vi "Arduino Find Home.vi"(7 "log ref":refnum<file>, 8 "error in":errorcluster, 9 "Homing Parameters":T1={"Direction (F: CW)"=FALSE, "Speed"=400, "Accel"=400, "Min Distance"=2700, "Short Leg"=0, "Error Cnts"=0}, 10 "Motor":i32, 11 "Addr":refnum<visa-resource-name>) -> (0 "error out":errorcluster, 2 "Success":bool, 3 "Log":string)   [LabVIEW 2021, in "FW Arduino Control.lvclass"]
uses:
  FW Arduino Control.lvclass
  Filter Wheel Arduino Homing cluster.ctl
panel:
  out "moves":i32
  out "Move distances":i32[](array[numeric])
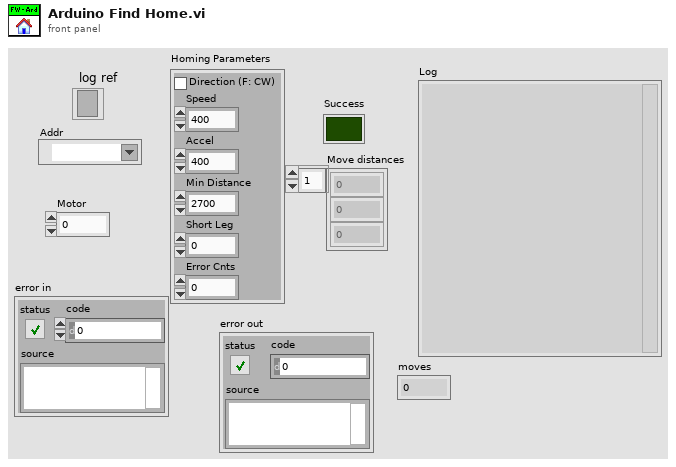
[diagram p1: front panel]
types:
  T1 = typedef "Filter Wheel Arduino Homing cluster.ctl" = cluster{"Direction (F: CW)":bool, "Speed":i32, "Accel":i32, "Min Distance":i32, "Short Leg":i32, "Error Cnts":i32}
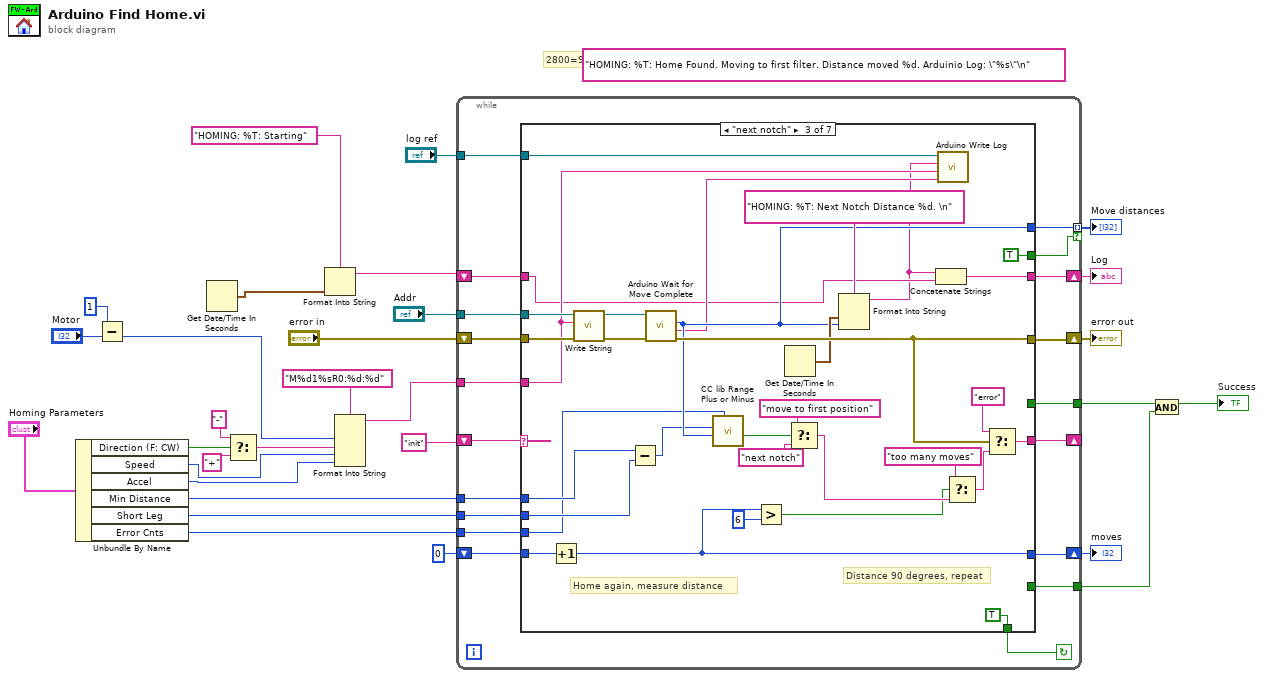
[diagram p0: block diagram]
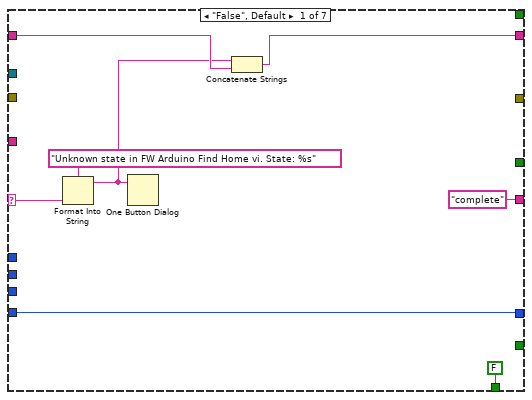
[diagram p2: hidden frame]
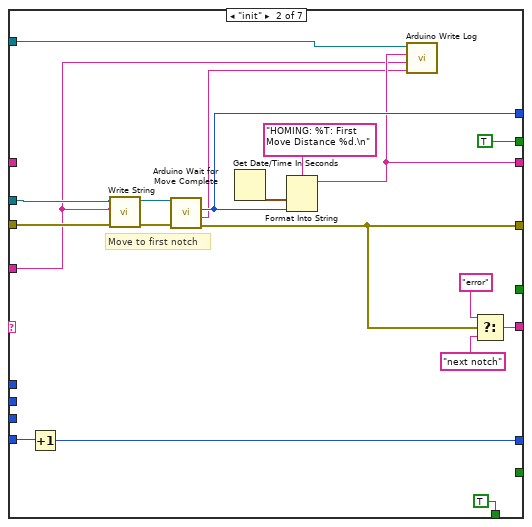
[diagram p3: hidden frame]
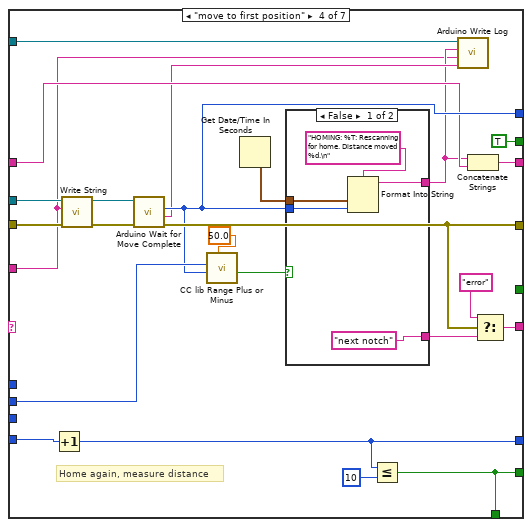
[diagram p4: hidden frame]
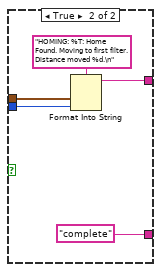
[diagram p5: hidden frame]
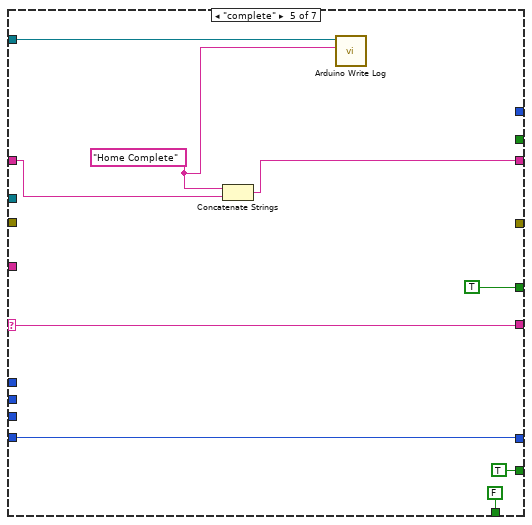
[diagram p6: hidden frame]
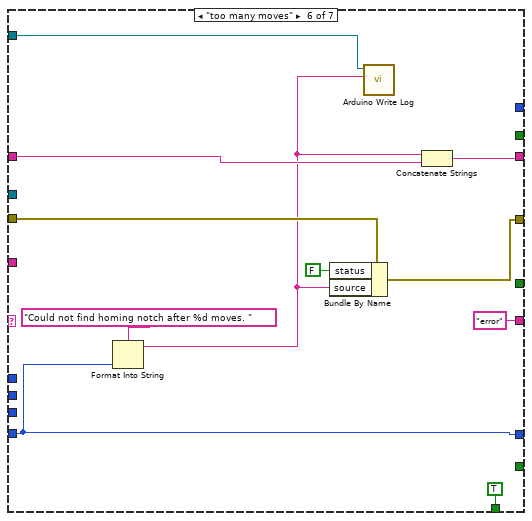
[diagram p7: hidden frame]
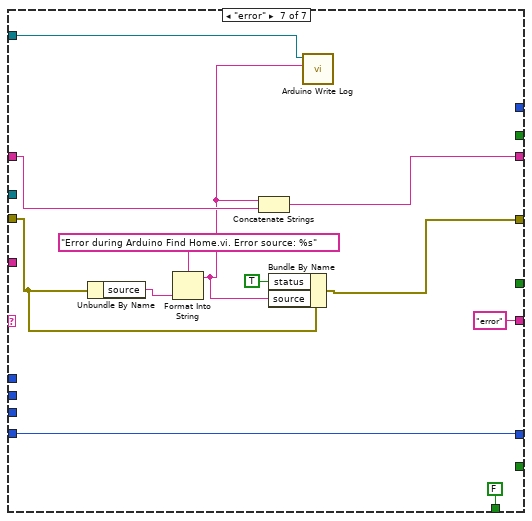
[diagram p8: hidden frame]
diagram:
  (unwired) "HOMING: %T: Home Found. Moving to first filter. Distance moved %d. Arduinio Log: \"%s\"\n" ("format string")
  # "2800=90degrees"
  n1 = Unbundle By Name("Homing Parameters") -> ("Direction (F: CW)"=w19:bool, "Speed"=w18:i32, "Accel"=w17:i32, "Min Distance"=w12:i32, "Short Leg"=w10:i32, "Error Cnts"=w1:i32)
  n2 = Subtract(x=1, y="Motor") -> (x-y=w3:i32)
  n3 = Get Date/Time In Seconds() -> (seconds since 1Jan1904=w14:timestamp)
  n4 = Select(t="-", s=w19, f="+") -> (s? t:f=w24:string)
  n5 = Format Into String(format string="HOMING: %T: Starting", w14) -> (resulting string=w13:string)  [unwired: 2 in, 1 out]
  n6 = Format Into String(format string="M%d1%sR0:%d:%d", w3, w24, w18, w17) -> (resulting string=w23:string)  [unwired: 2 in, 1 out]
  n7 = while {
    tunnel: "Addr" -> [w46]
    shift-right: [w47] -> _
    shift-left: "init" -> [w49]
    tunnel: w23 -> [w45]
    shift-right: [w44] -> w22
    shift-left: "error in" -> [w43]
    shift-right: [w42] -> w16
    shift-left: w13 -> [w41]
    tunnel: w12 -> [w40]
    tunnel: [w39] -> w11
    tunnel: w10 -> [w38]
    tunnel: [w37] -> w9 mode=indexing if=w36
    shift-right: [w34] -> w7
    shift-left: 0 -> [w35]
    tunnel: [w33] -> w5
    tunnel: "log ref" -> [w32]
    tunnel: w1 -> [w31]
    stop <- w48 continue-if-true
    n8 = case shown="\"next notch\"" w49 {
      selector: w49 -> [w56 _ _ _ w150 _ _]
      tunnel: [FALSE TRUE TRUE w115 FALSE TRUE FALSE] -> w48
      tunnel: ["complete" w73 w106 w131 w150 "error" "error"] -> w47
      tunnel: w46 -> [_ w71 w100 w127 _ _ _]
      tunnel: w45 -> [_ w58 w82 w109 _ _ _]
      tunnel: [_ w72 w103 w130 _ w155 w171] -> w44
      tunnel: w43 -> [_ w68 w99 w126 _ w162 w174]
      tunnel: [w51 w60 w80 w112 w148 w154 w163] -> w42
      tunnel: w41 -> [w53 _ w79 w113 w149 w160 w165]
      tunnel: w40 -> [_ _ w94 _ _ _ _]
      tunnel: [_ _ _ _ TRUE _ _] -> w39
      tunnel: w38 -> [_ _ w93 w120 _ _ _]
      tunnel: [_ w65 w92 w119 _ _ _] -> w37
      tunnel: [_ TRUE TRUE TRUE _ _ _] -> w36
      tunnel: w35 -> [w50 w63 w95 w122 w146 w158 w168]
      tunnel: [w50 w62 w86 w117 w146 w158 w168] -> w34
      tunnel: [_ _ _ w115 TRUE _ _] -> w33
      tunnel: w32 -> [_ w61 w83 w114 w144 w153 w167]
      tunnel: w31 -> [_ _ w77 _ _ _ _]
      frame "False", Default {
        n9 = Format Into String(format string="Unknown state in FW Arduino Find Home vi. State: %s", w56) -> (resulting string=w52:string)  [unwired: 2 in, 1 out]
        n10 = One Button Dialog(message=w52) -> ()  [unwired: 1 in, 1 out]
        n11 = Concatenate Strings(w52, w53) -> (w51:string)
      }
      frame "init" {
        # "Move to first notch"
        n12 = Increment(x=w63) -> (x+1=w62:i32)
        n13 = call "Write String.vi"("error in (no error)"=w68, "String"=w58, "VISA resource name"=w71) -> ("error out"=w69:errorcluster, "VISA resource name out"=w70:refnum<visa-resource-name>)  [unwired: 7 in]
        n14 = call "Arduino Wait for Move Complete.vi"("error in (no error)"=w69, "reference"=w70) -> ("error out"=w72:errorcluster, "response"=w59:string, "distance"=w65:i32)  [unwired: 6 in, 1 out]
        n15 = Get Date/Time In Seconds() -> (seconds since 1Jan1904=w66:timestamp)
        n16 = Format Into String(format string="HOMING: %T: First Move Distance %d.\n", w66, w65) -> (resulting string=w60:string)  [unwired: 2 in, 1 out]
        n17 = call "Arduino Write Log.vi"("Arduino data"=w59, "Command"=w58, "Message"=w60, "log ref"=w61) -> ()  [unwired: 8 in]
        n18 = Select(t="error", s=w72, f="next notch") -> (s? t:f=w73:string)
      }
      frame "next notch" {
        # "Distance 90 degrees, repeat"
        # "Home again, measure distance"
        n19 = Increment(x=w95) -> (x+1=w86:i32)
        n20 = call "Write String.vi"("error in (no error)"=w99, "String"=w82, "VISA resource name"=w100) -> ("error out"=w102:errorcluster, "VISA resource name out"=w101:refnum<visa-resource-name>)  [unwired: 7 in]
        n21 = Subtract(x=w94, y=w93) -> (x-y=w91:i32)
        n22 = call "Arduino Wait for Move Complete.vi"("error in (no error)"=w102, "reference"=w101) -> ("error out"=w103:errorcluster, "response"=w81:string, "distance"=w92:i32)  [unwired: 6 in, 1 out]
        n23 = call "CC lib Range Plus or Minus.vi"("+/- Range"=w77, "Value"=w92, "Target"=w91) -> ("In Range?"=w90:bool)  [unwired: 7 in, 1 out]
        n24 = Greater?(x=w86, y=6) -> (0:w84:bool)
        n25 = Get Date/Time In Seconds() -> (seconds since 1Jan1904=w97:timestamp)
        n26 = Select(t="move to first position", s=w90, f="next notch") -> (s? t:f=w88:string)
        n27 = Format Into String(format string="HOMING: %T: Next Notch Distance %d. \n", w97, w92) -> (resulting string=w78:string)  [unwired: 2 in, 1 out]
        n28 = Concatenate Strings(w78, w79) -> (w80:string)
        n29 = call "Arduino Write Log.vi"("Arduino data"=w81, "Command"=w82, "Message"=w78, "log ref"=w83) -> ()  [unwired: 8 in]
        n30 = Select(t="too many moves", s=w84, f=w88) -> (s? t:f=w104:string)
        n31 = Select(t="error", s=w103, f=w104) -> (s? t:f=w106:string)
      }
      frame "move to first position" {
        # "Home again, measure distance"
        n32 = Increment(x=w122) -> (x+1=w117:i32)
        n33 = call "Write String.vi"("error in (no error)"=w126, "String"=w109, "VISA resource name"=w127) -> ("error out"=w129:errorcluster, "VISA resource name out"=w128:refnum<visa-resource-name>)  [unwired: 7 in]
        n34 = call "Arduino Wait for Move Complete.vi"("error in (no error)"=w129, "reference"=w128) -> ("error out"=w130:errorcluster, "response"=w111:string, "distance"=w119:i32)  [unwired: 6 in, 1 out]
        n35 = call "CC lib Range Plus or Minus.vi"("+/- Range"=50.0, "Value"=w119, "Target"=w120) -> ("In Range?"=w118:bool)  [unwired: 7 in, 1 out]
        n36 = Get Date/Time In Seconds() -> (seconds since 1Jan1904=w125:timestamp)
        n37 = case shown="False" w118 {
          tunnel: [w137 w141] -> w110
          tunnel: w125 -> [w136 w140]
          tunnel: w119 -> [w135 w139]
          tunnel: ["next notch" "complete"] -> w124
          frame False {
            n38 = Format Into String(format string="HOMING: %T: Rescanning for home. Distance moved %d.\n", w136, w135) -> (resulting string=w137:string)  [unwired: 2 in, 1 out]
          }
          frame True {
            n39 = Format Into String(format string="HOMING: %T: Home Found. Moving to first filter. Distance moved %d.\n", w140, w139) -> (resulting string=w141:string)  [unwired: 2 in, 1 out]
          }
        }
        n40 = Less Or Equal?(x=w117, y=10) -> (x <= y?=w115:bool)
        n41 = call "Arduino Write Log.vi"("Arduino data"=w111, "Command"=w109, "Message"=w110, "log ref"=w114) -> ()  [unwired: 8 in]
        n42 = Concatenate Strings(w110, w113) -> (w112:string)
        n43 = Select(t="error", s=w130, f=w124) -> (s? t:f=w131:string)
      }
      frame "complete" {
        w143 = "Home Complete" ("string")
        n44 = Concatenate Strings(w143, w149) -> (w148:string)
        n45 = call "Arduino Write Log.vi"("Message"=w143, "log ref"=w144) -> ()  [unwired: 10 in]
      }
      frame "too many moves" {
        n46 = Format Into String(format string="Could not find homing notch after %d moves. " ("source"), w158) -> (resulting string=w152:string)  [unwired: 2 in, 1 out]
        n47 = Bundle By Name(cluster=w162, "status"=FALSE, "source"=w152) -> (w155:errorcluster)
        n48 = call "Arduino Write Log.vi"("Message"=w152, "log ref"=w153) -> ()  [unwired: 10 in]
        n49 = Concatenate Strings(w152, w160) -> (w154:string)
      }
      frame "error" {
        n50 = Unbundle By Name(w174) -> ("source"=w173:string)
        n51 = Format Into String(format string="Error during Arduino Find Home.vi. Error source: %s", w173) -> (resulting string=w164:string)  [unwired: 2 in, 1 out]
        n52 = Concatenate Strings(w164, w165) -> (w163:string)
        n53 = Bundle By Name(cluster=w174, "status"=TRUE, "source"=w164) -> (w171:errorcluster)
        n54 = call "Arduino Write Log.vi"("Message"=w164, "log ref"=w167) -> ()  [unwired: 10 in]
      }
    }
  }
  "error out" <- w22
  "Log" <- w16
  "Move distances" <- w9
  "moves" <- w7
  n55 = And(x=w11, y=w5) -> (x .and. y?=→"Success":bool)
